vi "Main.vi"() -> ()   [LabVIEW 2015]
doc: "This template is for the Queued Message Handler design pattern.\n\nThe Event Handling Loop generates messages based on user interface actions.\n\nThe Message Handling Loop processes messages generated by the Event Handling Loop, or by other messages. The messages are string values, so new messages can be added easily to the Message Cases case structure in the Message Handling Loop. Each message cluster can also provide an optional value for Message Data, which is a variant that can be converted to whatever message-specific data is required."
uses:
  support/Type Definitions/UI Data.ctl
  support/Status Logger/Status Log.ctl
  <vilib>/Utility/error.llb/DialogType.ctl
  DAQ/TypeDefs/DAQ data.ctl
  support/Message Queue/Enqueue Message (Single).vi
  support/Global names.vi
  <vilib>/Utility/error.llb/Error Cluster From Error Code.vi
  <vilib>/ErrorRing/Error Ring.xnode
  support/Message Queue/Message Queue.lvlib
  Support/User Event - EHL Stop/User Event - EHL Stop.lvlib
  Model/Model.lvlib
  DAQ/DAQ.lvlib
  PLC/PLC.lvlib
panel:
  out "Power status":bool
  in  "Remote":bool
  in  "Abort":bool
  in  "Stop Line":bool
  in  "Start Line":bool
  out "Status":string
  in  "Tab Control":T1(tab)
  in  "Power switch":bool
  in  "Positon":dbl(slide) scale=0.0..20.0
  in  "Dispose":bool
  in  "Pump":bool
  in  "Flow [l/s]":dbl=10.0
  in  "Potentiometer (AI)":tag
  in  "LED (DO)":tag
  in  "Bistable switch (DI)":tag
  in  "Monostable switch (DI)":tag
  in  "Send":bool
  in  "Data to send":string
  out "Data received":string
  in  "Disconnect":bool
  in  "Connect":bool
  out "Connected?":bool
  in  "Type":enum16{"Server", "Client"}(ring)
  in  "Port":u16
  in  "IP":string
  in  "Current printer":u16(ring) items=["PDFCreator", "OKI DATA CORP C5950 kolor (C-2 218)", "Microsoft XPS Document Writer", "Microsoft Print to PDF", "HP LaserJet Professional P1606dn B&W (M3)", "hp LaserJet 1320 PCL 5 B&W (C-2 307)", "Fax", "Canon MP560 KOLOR (DOM)", "Brother PC-FAX v.3.2", "Brother MFC-L8850CDW KOLOR (M6)", "Brother MFC-L2740DW B&W (M6)", "Brother MFC-L2740DW B&W (M3)", "Brother DCP-9020CDW (Dziekan)"]
  in  "Check printers":bool
  in  "Print report":bool
  in  "TDMS View":bool
  in  "Exit":bool
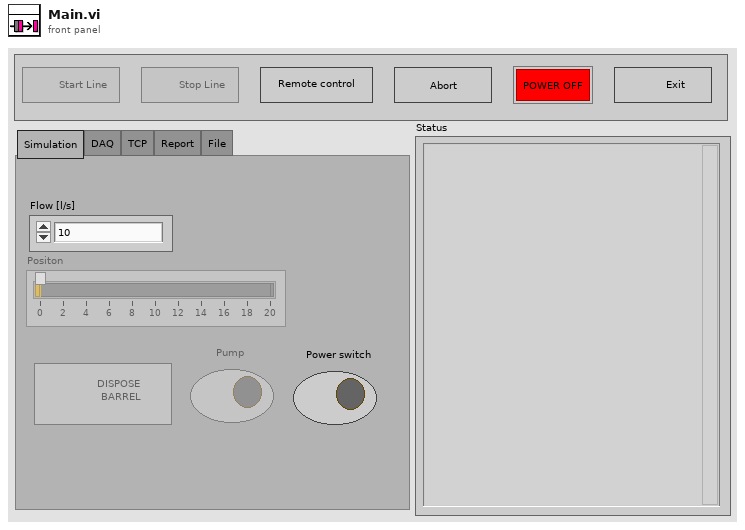
[diagram p1: front panel]
types:
  T1 = enum32{"Simulation", "DAQ", "TCP", "Report", "File"}
  T2 = typedef "Status Log.ctl" = enum16{"Close file", "Open Status file", "Add Status", "Show Status File"}
  T3 = typedef "UI Data.ctl" = cluster{"Start Line Ref":refnum<vi>, "Stop Line Ref":refnum<vi>, "Data Display Ref":refnum<vi>, "Exit Button Ref":refnum<vi>, "Pump Ref":refnum<vi>, "Dispose Ref":refnum<vi>, "Flow Ref":refnum<vi>, "Position Ref":refnum<vi>, "Tab Ref":refnum<vi>, "Print report":refnum<vi>, "Remote":refnum<vi>, "Connection status":refnum<vi>, "Abort":refnum<vi>, "Power status":refnum<vi>, "Power switch":refnum<vi>}
  T4 = typedef "Notifiers.lvlib/Notifiers.ctl" = cluster{"PLC":refnum<notifier>, "Model":refnum<notifier>, "DAQ":refnum<notifier>}
  T5 = typedef "Message Queue.lvlib/All Message Queues.ctl" = cluster{"UI":refnum<queue>, "Model":refnum<queue>, "DAQ":refnum<queue>, "PLC":refnum<queue>}
  T6 = typedef "DialogType.ctl" = u16
  T7 = typedef "DAQ.lvlib/DAQ data.ctl" = cluster{"Power switch (DI)":cluster{"Channel":tag, "Data":bool}, "Dispose barrel (DI)":cluster{"Channel":tag, "Data":bool}, "Pump status (DO)":cluster{"Channel":tag, "Data":bool}, "Barrel position (AI)":cluster{"Channel":tag, "Data":dbl}}
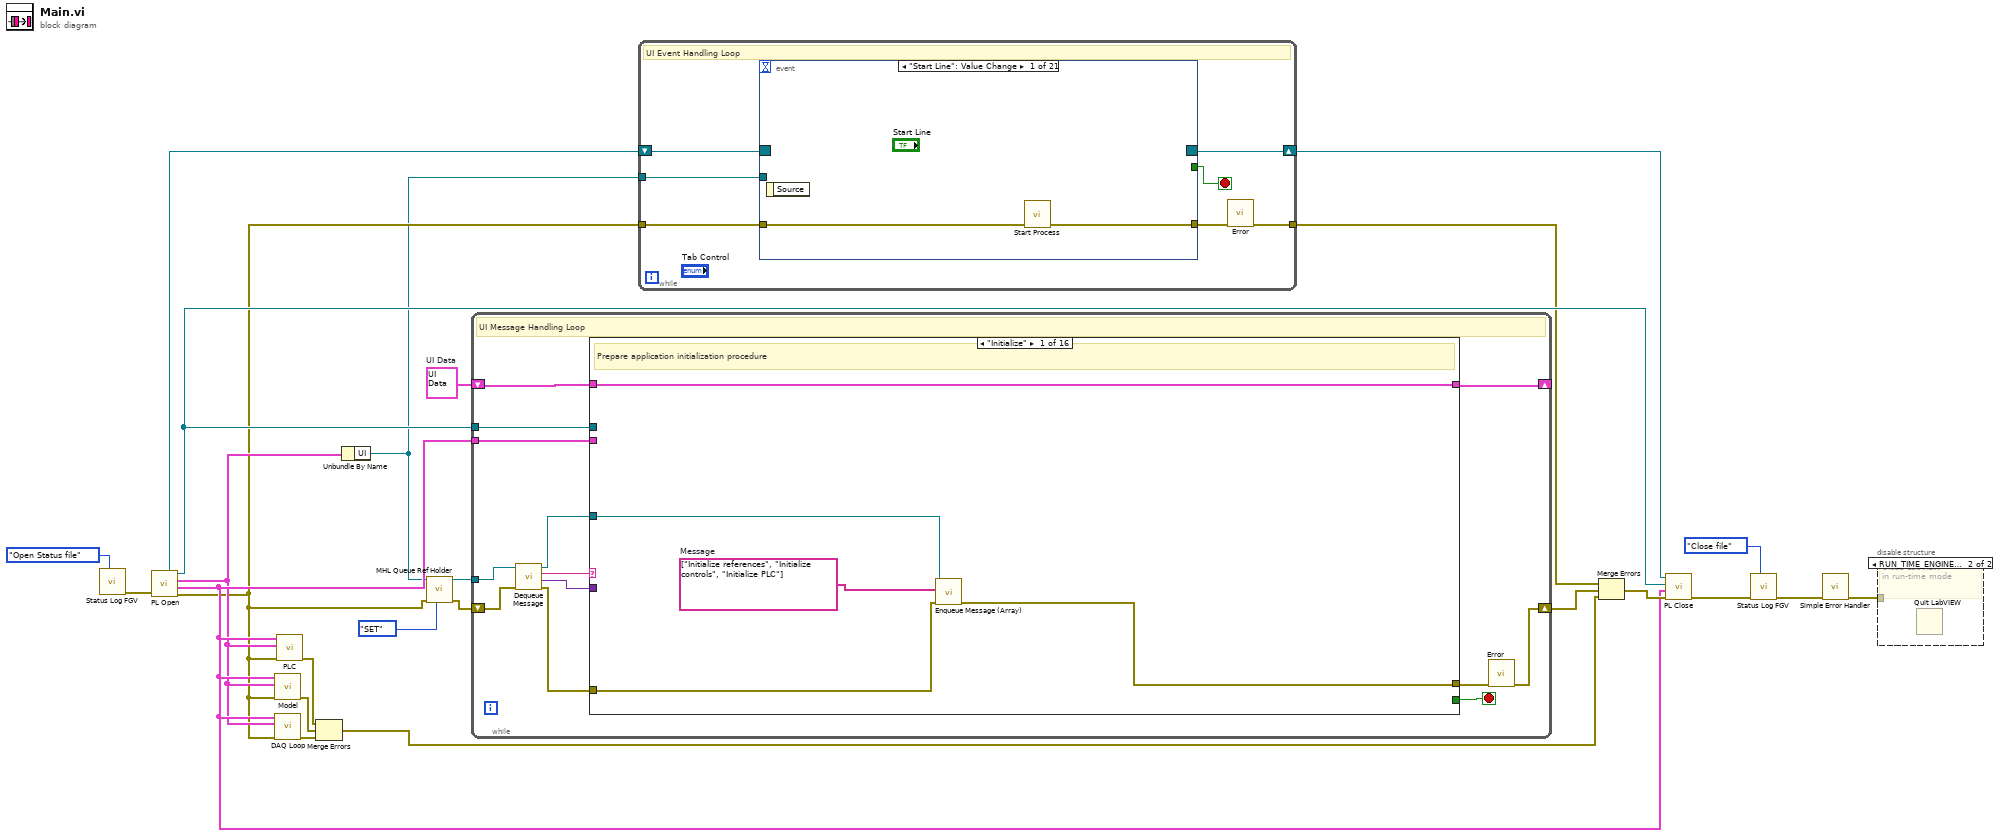
[diagram p0: block diagram]
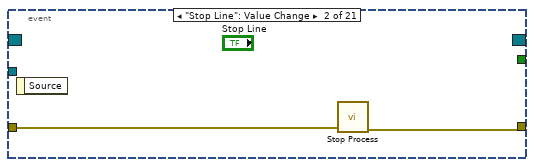
[diagram p2: hidden frame]
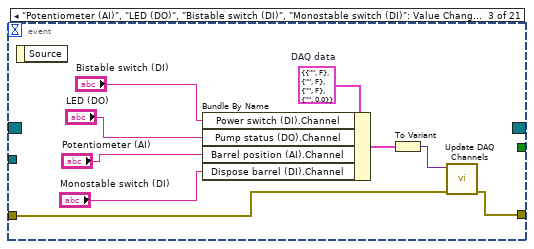
[diagram p3: hidden frame]
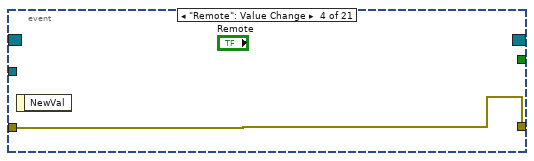
[diagram p4: hidden frame]
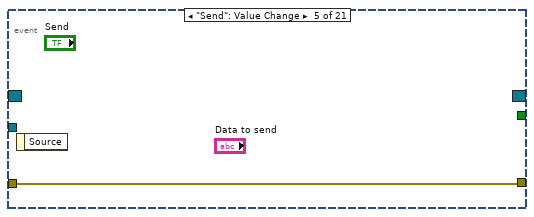
[diagram p5: hidden frame]
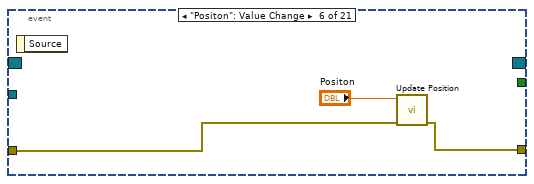
[diagram p6: hidden frame]
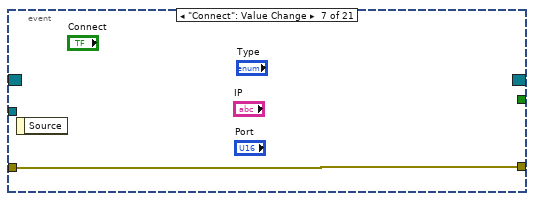
[diagram p7: hidden frame]
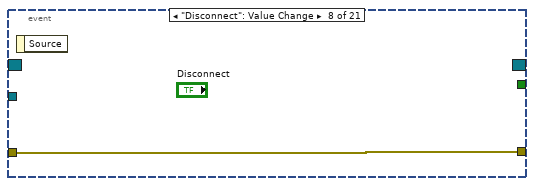
[diagram p8: hidden frame]
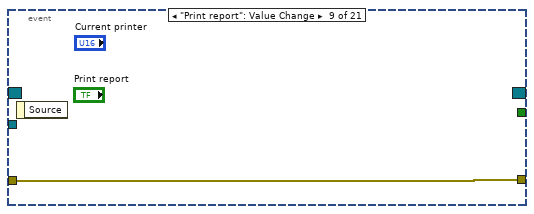
[diagram p9: hidden frame]
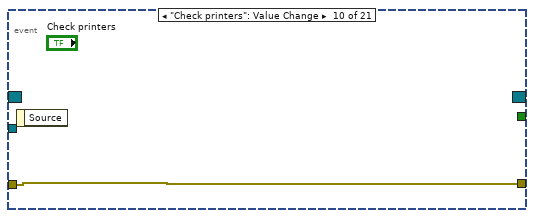
[diagram p10: hidden frame]
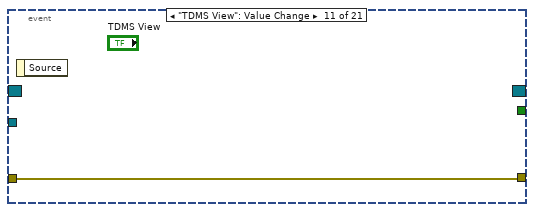
[diagram p11: hidden frame]
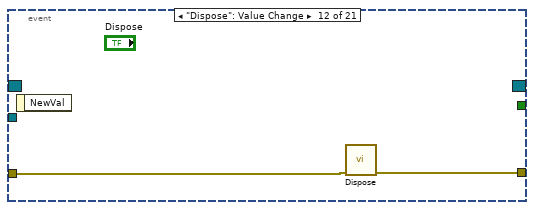
[diagram p12: hidden frame]
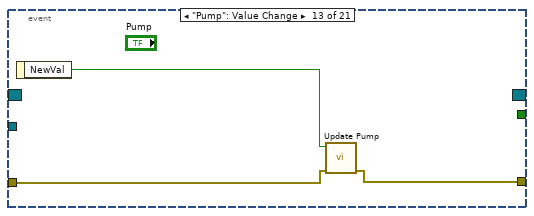
[diagram p13: hidden frame]
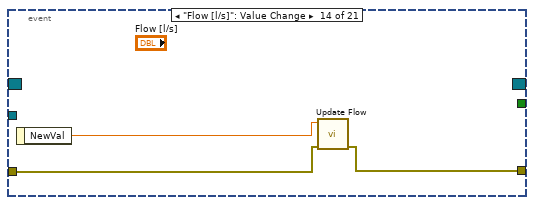
[diagram p14: hidden frame]
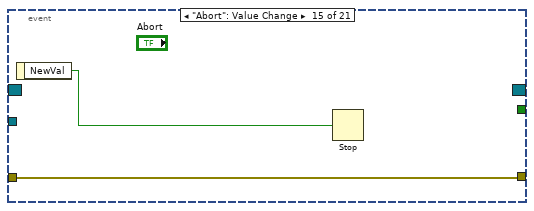
[diagram p15: hidden frame]
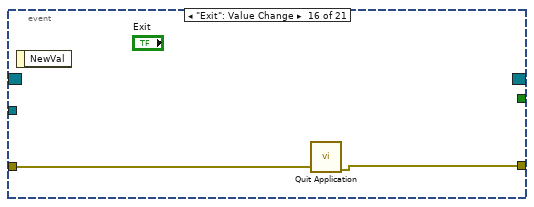
[diagram p16: hidden frame]
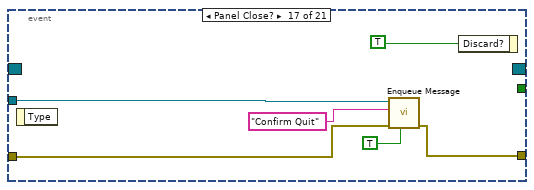
[diagram p17: hidden frame]
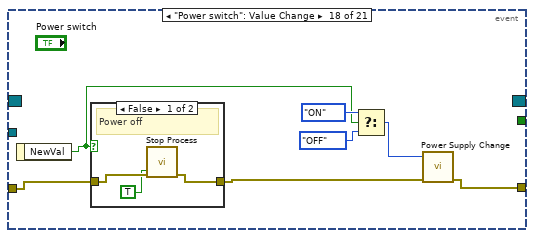
[diagram p18: hidden frame]
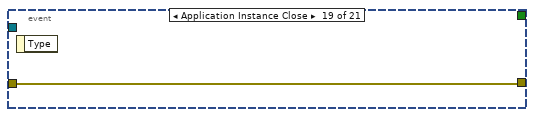
[diagram p20: hidden frame]
diagram:
  w23 = T3 {"Start Line Ref"=refnum, "Stop Line Ref"=refnum, "Data Display Ref"=refnum, "Exit Button Ref"=refnum, "Pump Ref"=refnum, "Dispose Ref"=refnum, "Flow Ref"=refnum, "Position Ref"=refnum, "Tab Ref"=refnum, "Print report"=refnum, "Remote"=refnum, "Connection status"=refnum, "Abort"=refnum, "Power status"=refnum, "Power switch"=refnum}  # UI Data
  n1 = call "Status Log FGV.vi"("Action"=Status_Log."Open Status file") -> ("error out"=w18:errorcluster)  [unwired: 10 in]
  n2 = call "PL Open.vi"("error in"=w18) -> ("error out"=w4:errorcluster, "Notifiers"=w11:T4, "Queues"=w10:T5, "User Event"=w21:refnum<user-event>, "Event Registration Refnum"=w13:refnum<event-registration>)  [unwired: 6 in]
  n3 = call "Model.vi"("error in"=w4, "Queues"=w10, "Notifiers"=w11) -> ("error out"=w8:errorcluster)  [unwired: 8 in]
  n4 = call "DAQ Loop.vi"("error in"=w4, "Queues"=w10, "Notifiers"=w11) -> ("error out"=w7:errorcluster)  [unwired: 8 in]
  n5 = call "PLC.vi"("error in"=w4, "Message Queues"=w10, "Notifiers"=w11) -> ("error out"=w9:errorcluster)  [unwired: 8 in]
  n6 = Merge Errors(w9, w8, w7) -> (w6:errorcluster)
  n7 = Unbundle By Name(w10) -> ("UI"=w1:refnum<queue>)
  n8 = call "MHL Queue Ref Holder.vi"("Action"=enum16{"GET", "SET"}."SET", "error in"=w4, "Message Queue In"=w1) -> ("error out"=w3:errorcluster, "Input Message Queue"=w5:refnum<queue>)  [unwired: 7 in]
  n9 = while {
    shift-right: [w36] -> _
    shift-left: w23 -> [w37]
    tunnel: w21 -> [w34]
    tunnel: w11 -> [w30]
    shift-right: [w26] -> w17
    shift-left: w3 -> [w33]
    tunnel: w5 -> [w28]
    stop <- w35 stop-if-true
    # "UI Message Handling Loop"
    n10 = call "Dequeue Message.vi"("error in (no error)"=w33, "Message Queue"=w28) -> ("error out"=w32:errorcluster, "Message Data"=w29:variant, "Message"=w25:string, "dup Message Queue"=w31:refnum<queue>)  [unwired: 6 in]
    n11 = case "Message Cases" shown="\"Initialize\"" w25 {
      selector: w25 -> [_ _ _ _ _ _ _ _ _ _ _ _ _ _ _ w268]
      tunnel: w31 -> [w39 _ _ _ _ _ _ _ _ _ _ w214 w220 w256 _ _]
      tunnel: w32 -> [w40 w46 w69 w103 w118 w137 w151 w167 w174 w203 w206 w215 w222 w239 w263 _]
      tunnel: [w38 w46 w78 w104 w117 w139 w152 w168 w174 w199 w205 w212 w219 w243 w257 w267] -> w27
      tunnel: w37 -> [w41 w60 w89 w105 w124 w149 w158 w171 w175 w181 w210 w216 w226 w248 w262 w269]
      tunnel: [w41 w47 w89 w105 w124 w149 w158 w171 w175 w181 w210 w216 w226 w248 w262 w269] -> w36
      tunnel: [_ _ _ _ _ _ _ _ _ _ _ _ _ TRUE _ _] -> w35
      tunnel: w29 -> [_ _ _ _ _ _ w162 w165 _ w202 w209 _ _ w250 _ _]
      tunnel: w34 -> [_ _ _ _ _ _ _ _ _ _ _ _ _ w253 _ _]
      tunnel: w30 -> [_ _ _ _ _ _ _ _ _ _ _ _ w225 _ _ _]
      frame "Initialize" {
        w42 = string[] ["Initialize references", "Initialize controls", "Initialize PLC"]  # Message
        # "Prepare application initialization procedure"
        n12 = call "Enqueue Message (Array).vi"("error in (no error)"=w40, "Message Array"=w42, "Message Queue"=w39) -> ("error out"=w38:errorcluster)  [unwired: 7 in, 1 out]
      }
      frame "Initialize references" {
        # "Link references to UI objects"
        n13 = control-ref of="Power switch"() -> (w43:refnum<vi>)
        n14 = control-ref of="Stop Line"() -> (w57:refnum<vi>)
        n15 = control-ref of="Flow [l/s]"() -> (w54:refnum<vi>)
        n16 = control-ref of="Dispose"() -> (w55:refnum<vi>)
        n17 = control-ref of="Exit"() -> (w59:refnum<vi>)
        n18 = control-ref of="Start Line"() -> (w58:refnum<vi>)
        n19 = control-ref of="Pump"() -> (w56:refnum<vi>)
        n20 = Bundle By Name(cluster=w60, "Exit Button Ref"=w59, "Start Line Ref"=w58, "Stop Line Ref"=w57, "Pump Ref"=w56, "Dispose Ref"=w55, "Flow Ref"=w54, "Power switch"=w43) -> (w53:T3)
        n21 = control-ref of="Tab Control"() -> (w51:refnum<vi>)
        n22 = control-ref of="Remote"() -> (w49:refnum<vi>)
        n23 = control-ref of="Connection status"() -> (w48:refnum<vi>)
        n24 = control-ref of="Positon"() -> (w52:refnum<vi>)
        n25 = control-ref of="Print report"() -> (w50:refnum<vi>)
        n26 = control-ref of="Power status"() -> (w44:refnum<vi>)
        n27 = control-ref of="Abort"() -> (w45:refnum<vi>)
        n28 = Bundle By Name(cluster=w53, "Position Ref"=w52, "Tab Ref"=w51, "Print report"=w50, "Remote"=w49, "Connection status"=w48, "Abort"=w45, "Power status"=w44) -> (w47:T3)
      }
      frame "Initialize controls" {
        w61 = TRUE ("Enabled")
        w62 = FALSE ("Enabled")
        # "Initialize activity and values of UI objects"
        n29 = Unbundle By Name(w89) -> ("Stop Line Ref"=w102:refnum<vi>, "Print report"=w84:refnum<vi>)
        n30 = Current VI's Menubar() -> (w64:refnum<k9>)
        n31 = Build Array(w102, w84) -> (w101:refnum<vi>[])
        n32 = call "Enable Multiple Controls.vi"("error in"=w69, "Enabled"=w62, "References"=w101) -> ("error out"=w98:errorcluster)  [unwired: 8 in]
        n33 = Set Menu Item Info(7:"Stop" ("item tag"), 8:w69, 9:w62, 11:w64) -> (0:w67:errorcluster, 3:w63:refnum<k9>)  [unwired: 3 in]
        n34 = Unbundle By Name(w89) -> ("Exit Button Ref"=w100:refnum<vi>, "Start Line Ref"=w99:refnum<vi>)
        n35 = call "Power Supply Change.vi"("error in"=w69, "Power status"=enum16{"OFF", "ON"}."OFF") -> ("error out"=w75:errorcluster)  [unwired: 9 in]
        n36 = Build Array(w100, w99) -> (w97:refnum<vi>[])
        n37 = call "Enable Multiple Controls.vi"("error in"=w98, "Enabled"=w61, "References"=w97) -> ("error out"=w92:errorcluster)  [unwired: 8 in]
        n38 = Set Menu Item Info(7:"Start" ("item tag"), 8:w67, 9:w61, 11:w63) -> (0:w65:errorcluster)  [unwired: 3 in, 1 out]
        n39 = Unbundle By Name(w89) -> ("Exit Button Ref"=w96:refnum<vi>, "Start Line Ref"=w95:refnum<vi>, "Stop Line Ref"=w94:refnum<vi>, "Pump Ref"=w93:refnum<vi>, "Remote"=w83:refnum<vi>, "Connection status"=w82:refnum<vi>, "Abort"=w81:refnum<vi>, "Power status"=w80:refnum<vi>, "Power switch"=w71:refnum<vi>)
        n40 = call "Status Display.vi"("Action"=enum16{"Update", "Clear"}."Clear", "error in"=w75) -> ("error out"=w74:errorcluster, "Status"=w72:string)  [unwired: 8 in]
        n41 = local write "Status"(w72) -> ()
        n42 = Build Array(w96, w95, w94, w93, w83, w82, w81, w80, w71) -> (w90:refnum<vi>[])
        n43 = call "Value Multiple Boolean Controls.vi"("error in"=w92, "Value"=FALSE ("Enabled"), "References"=w90) -> ("error out"=w88:errorcluster)  [unwired: 8 in]
        n44 = Unbundle By Name(w89) -> ("Position Ref"=w87:refnum<vi>)
        n45 = Build Array(w87) -> (w86:refnum<vi>[])
        n46 = call "Value Multiple Numeric Controls.vi"("error in"=w88, "Value"=0.0, "References"=w86) -> ("error out"=w77:errorcluster)  [unwired: 8 in]
        n47 = call "Update Display.vi"("error in"=w77, "Message string"="UI initialized") -> ("error out"=w66:errorcluster)  [unwired: 9 in]
        n48 = Merge Errors(w66, w65, w74) -> (w78:errorcluster)
      }
      frame "Initialize PLC" {
        # "Initialize Production Line Controller"
        n49 = call "Initialize.vi"("error in"=w103) -> ("error out"=w104:errorcluster)  [unwired: 10 in]
      }
      frame "Start process" {
        w109 = TRUE ("Enabled")
        w113 = FALSE ("Enabled")
        # "Starts process: start PLC, open logger file, create reports files, enable/disable UI controls and update status display"
        n50 = Unbundle By Name(w124) -> ("Exit Button Ref"=w106:refnum<vi>, "Start Line Ref"=w119:refnum<vi>, "Stop Line Ref"=w123:refnum<vi>)
        n51 = Build Array(w106, w119) -> (w125:refnum<vi>[])
        n52 = Build Array(w123) -> (w122:refnum<vi>[])
        n53 = call "Start.vi"("error in"=w118) -> ("error out"=w121:errorcluster)  [unwired: 10 in]
        n54 = call "Enable Multiple Controls.vi"("error in"=w118, "Enabled"=w109, "References"=w122) -> ("error out"=w111:errorcluster)  [unwired: 8 in]
        n55 = call "Enable Multiple Controls.vi"("error in"=w118, "Enabled"=w113, "References"=w125) -> ("error out"=w115:errorcluster)  [unwired: 8 in]
        n56 = global read "Global names.vi" "Starting"() -> (w107:string)
        n57 = Current VI's Menubar() -> (w108:refnum<k9>)
        n58 = call "Update Display.vi"("error in"=w121, "Message string"=w107) -> ("error out"=w120:errorcluster)  [unwired: 9 in]
        n59 = Set Menu Item Info(7:"Start" ("item tag"), 8:w115, 9:w113, 11:w108) -> (0:w114:errorcluster)  [unwired: 3 in, 1 out]
        n60 = Set Menu Item Info(7:"Stop" ("item tag"), 8:w111, 9:w109, 11:w108) -> (0:w110:errorcluster)  [unwired: 3 in, 1 out]
        n61 = Merge Errors(w120, w114, w110) -> (w117:errorcluster)
      }
      frame "Stop process" {
        w128 = FALSE ("Enabled")
        w129 = TRUE ("Enabled")
        # "Stops process: stop PLC, close logger file, save and close report files, enable/disable UI controls and update status display"
        n62 = Unbundle By Name(w149) -> ("Exit Button Ref"=w126:refnum<vi>, "Start Line Ref"=w142:refnum<vi>, "Stop Line Ref"=w148:refnum<vi>)
        n63 = call "Stop.vi"("error in"=w137) -> ("error out"=w144:errorcluster)  [unwired: 10 in]
        n64 = Build Array(w148) -> (w138:refnum<vi>[])
        n65 = Build Array(w126, w142) -> (w146:refnum<vi>[])
        n66 = global read "Global names.vi" "Stopping"() -> (w127:string)
        n67 = Build Array (concatenate)(w146, w138) -> (w145:refnum<vi>[])
        n68 = call "Enable Multiple Controls.vi"("error in"=w137, "Enabled"=w129, "References"=w146) -> ("error out"=w134:errorcluster)  [unwired: 8 in]
        n69 = call "Enable Multiple Controls.vi"("error in"=w137, "Enabled"=w128, "References"=w138) -> ("error out"=w141:errorcluster)  [unwired: 8 in]
        n70 = call "Value Multiple Boolean Controls.vi"("error in"=w137, "Value"=FALSE, "References"=w145) -> ("error out"=w140:errorcluster)  [unwired: 8 in]
        n71 = call "Update Display.vi"("error in"=w144, "Message string"=w127) -> ("error out"=w143:errorcluster)  [unwired: 9 in]
        n72 = Current VI's Menubar() -> (w135:refnum<k9>)
        n73 = Set Menu Item Info(7:"Start" ("item tag"), 8:w134, 9:w129, 11:w135) -> (0:w132:errorcluster, 3:w130:refnum<k9>)  [unwired: 3 in]
        n74 = Set Menu Item Info(7:"Stop" ("item tag"), 8:w132, 9:w128, 11:w130) -> (0:w131:errorcluster)  [unwired: 3 in, 1 out]
        n75 = Merge Errors(w143, w131, w141, w140) -> (w139:errorcluster)
      }
      frame "Update display" {
        # "Updates status display, status log file and word report file"
        n76 = Variant To Data(error in=w151, type="", Variant=w162) -> (data=w150:string, error out=w155:errorcluster)
        n77 = call "Status Display.vi"("Action"=enum16{"Update", "Clear"}."Update", "error in"=w155, "Status line"=w150) -> ("error out"=w153:errorcluster, "Status"=→"Status":string)  [unwired: 7 in]
        n78 = call "Status Log FGV.vi"("Action"=Status_Log."Add Status", "error in"=w155, "Status"=w150) -> ("error out"=w154:errorcluster)  [unwired: 8 in]
        n79 = property on="Status" class="Str"("Text.Scroll Position"=-1) -> ()  [unwired: 2 in, 2 out]
        n80 = Merge Errors(w154, w153) -> (w152:errorcluster)
      }
      frame "Update position" {
        # "Programmatically update position of the barrel slider"
        n81 = Variant To Data(error in=w167, type=0.0 ("Value"), Variant=w165) -> (data=w163:dbl, error out=w166:errorcluster)
        n82 = Unbundle By Name(w171) -> ("Position Ref"=w170:refnum<vi>)
        n83 = Build Array(w170) -> (w169:refnum<vi>[])
        n84 = call "Value Multiple Numeric Controls.vi"("error in"=w166, "Value"=w163, "References"=w169) -> ("error out"=w168:errorcluster)  [unwired: 8 in]
      }
      frame "Update Connection UI" {
        # "Updates TCP conection UI indicators"
        "Data received" <- "" ("Data received")
        "Connected?" <- FALSE ("Connected?")
      }
      frame "Power status change" {
        # "Update main switch LED and Start/Stop buttons according to power status change (DAQ DI)"
        n85 = Variant To Data(error in=w203, type=TRUE, Variant=w202) -> (data=w182:bool, error out=w186:errorcluster)
        "Power status" <- w182
        n86 = Unbundle By Name(w181) -> ("Position Ref"=w176:refnum<vi>, "Dispose Ref"=w180:refnum<vi>, "Pump Ref"=w179:refnum<vi>)
        n87 = Unbundle By Name(w181) -> ("Start Line Ref"=w178:refnum<vi>, "Stop Line Ref"=w200:refnum<vi>)
        n88 = Build Array(w176, w180, w179, w178) -> (w177:refnum<vi>[])
        n89 = Build Array(w178) -> (w198:refnum<vi>[])
        n90 = Build Array(w200) -> (w195:refnum<vi>[])
        n91 = Build Array (concatenate)(w198, w195) -> (w197:refnum<vi>[])
        n92 = Current VI's Menubar() -> (w189:refnum<k9>)
        n93 = call "Enable Multiple Controls.vi"("error in"=w186, "Enabled"=w182, "References"=w177) -> ("error out"=w193:errorcluster)  [unwired: 8 in]
        n94 = Set Menu Item Info(7:"Start" ("item tag"), 8:w186, 9:w182, 11:w189) -> (0:w187:errorcluster, 3:w183:refnum<k9>)  [unwired: 3 in]
        n95 = call "Value Multiple Boolean Controls.vi"("error in"=w186, "Value"=FALSE, "References"=w197) -> ("error out"=w192:errorcluster)  [unwired: 8 in]
        n96 = call "Enable Multiple Controls.vi"("error in"=w186, "Enabled"=FALSE, "References"=w195) -> ("error out"=w191:errorcluster)  [unwired: 8 in]
        n97 = Set Menu Item Info(7:"Stop" ("item tag"), 8:w187, 9:FALSE ("enabled"), 11:w183) -> (0:w184:errorcluster)  [unwired: 3 in, 1 out]
        n98 = Merge Errors(w193, w192, w191, w184) -> (w199:errorcluster)
      }
      frame "Error" {
        w204 = T6 2 items=["no dialog", "OK message", "continue or stop message", "OK message + warnings", "continue/stop + warnings"] ("type of dialog (OK msg:1)")
        # "Display error dialog box and quit application"
        n99 = Variant To Data(error in=w206, type=errorcluster {"status"=FALSE, "code"=0, "source"=""} ("error constant"), Variant=w209) -> (data=w207:errorcluster, error out=w205:errorcluster)
        n100 = call <vilib>:"Simple Error Handler.vi"("type of dialog (OK msg:1)"=w204, "error in (no error)"=w207) -> ()  [unwired: 3 in, 5 out]
      }
      frame "Exit" {
        # "Start exit procedure: stop PLC, then send Exit message to PLC and go to PLC confirmation loop"
        n101 = Flush Queue(queue=w214, error in (no error)=w215) -> (error out=w211:errorcluster)  [unwired: 2 out]
        n102 = call "Exit PLC.vi"("error in"=w211) -> ("error out"=w213:errorcluster)  [unwired: 10 in]
        n103 = call "Wait on PLC Exit.vi"("error in"=w213) -> ("error out"=w212:errorcluster)  [unwired: 10 in]
      }
      frame "Wait on PLC exit" {
        # "Wait until PLC shutdown"
        n104 = Unbundle By Name(w225) -> ("PLC"=w224:refnum<notifier>)
        n105 = Wait on Notification(notifier=w224, timeout in ms (-1)=10, error in (no error)=w222) -> (notification=w218:string, timed out?=w221:bool, error out=w217:errorcluster)  [unwired: 1 in, 1 out]
        n106 = case shown="True" w221 {
          tunnel: [w227 w236] -> w219
          tunnel: w217 -> [w228 w233]
          tunnel: w220 -> [_ w234]
          tunnel: w218 -> [_ w229]
          frame True {
            # "Shutdown notification from PLC not received"
            n107 = call "Wait on PLC Exit.vi"("error in"=w228) -> ("error out"=w227:errorcluster)  [unwired: 10 in]
          }
          frame False {
            # "Shutdown notification from PLC received (handshake)"
            n108 = call "Update Display.vi"("error in"=w233, "Message string"=w229) -> ("error out"=w232:errorcluster)  [unwired: 9 in]
            n109 = call "Update Display.vi"("error in"=w232, "Message string"="Application quits" ("Message")) -> ("error out"=w231:errorcluster)  [unwired: 9 in]
            n110 = call-poly "Enqueue Message.vi"("error in (no error)"=w231, "Message"="End program", "Message Queue"=w234) -> ("error out"=w236:errorcluster)  [unwired: 7 in, 1 out]
          }
        }
      }
      frame "End program" {
        # "Shutdown MHL and send exit user event to EHL; reset UI controls"
        n111 = call "Fire User Event - EHL Stop.vi"("error in (no error)"=w239, "User Event - Stop"=w253) -> ("error out"=w238:errorcluster)  [unwired: 9 in]
        n112 = Variant To Data(error in=w239, type=errorcluster {"status"=FALSE, "code"=0, "source"=""} ("error constant"), Variant=w250) -> (data=w251:errorcluster)  [unwired: 1 out]
        n113 = Release Queue(queue=w256, force destroy? (F)=TRUE, error in (no error)=w239) -> (error out=w254:errorcluster)  [unwired: 2 out]
        n114 = call <vilib>:"Simple Error Handler.vi"("error in (no error)"=w251) -> ("error out"=w237:errorcluster)  [unwired: 4 in, 4 out]
        n115 = Merge Errors(w238, w237, w254) -> (w244:errorcluster)
        n116 = Unbundle By Name(w248) -> ("Exit Button Ref"=w247:refnum<vi>, "Abort"=w242:refnum<vi>, "Start Line Ref"=w241:refnum<vi>, "Stop Line Ref"=w240:refnum<vi>)
        n117 = Build Array(w247, w242, w241, w240) -> (w246:refnum<vi>[])
        n118 = call "Value Multiple Boolean Controls.vi"("error in"=w244, "Value"=FALSE, "References"=w246) -> ("error out"=w243:errorcluster)  [unwired: 8 in]
      }
      frame "Confirm Quit" {
        # "Confirm Quit - Message that can confirm whether or not the user wants to exit the application."
        n119 = Two Button Dialog(message="Are you sure?", 1:"Continue" ("F button name (\"Cancel\")"), 2:"Quit" ("T button name (\"OK\")")) -> (T button?=w258:bool)
        n120 = case shown="True" w258 {
          tunnel: w263 -> [w264 w266]
          tunnel: [w264 w265] -> w257
          frame False {
          }
          frame True {
            n121 = call "Quit Application.vi"("error in"=w266) -> ("error out"=w265:errorcluster)  [unwired: 10 in]
          }
        }
      }
      frame Default {
        # "Incorrect message: show error and clear error"
        n122 = xnode "Error Ring"("parameter 0"=w268) -> ("error out"=w267:errorcluster)
      }
    }
    n123 = call "Error.vi"("error in"=w27) -> ("error out"=w26:errorcluster)  [unwired: 10 in]
  }
  n124 = while {
    tunnel: w1 -> [w279]
    shift-right: [w282] -> w24
    shift-left: w13 -> [w283]
    tunnel: [w277] -> w12
    tunnel: w4 -> [w280]
    stop <- w281 stop-if-true
    # "UI Event Handling Loop"
    n125 = event shown="[0] \"Start Line\": Value Change" {
      selector: w283 -> [_ _ _ _ _ _ _ _ _ _ _ _ _ _ _ _ _ _ _ _ _]
      dyn-events: [_ _ _ _ _ _ _ _ _ _ _ _ _ _ _ _ _ _ _ _ _] -> w282
      timeout: _ -> [_ _ _ _ _ _ _ _ _ _ _ _ _ _ _ _ _ _ _ _ _]
      tunnel: [_ _ _ _ _ _ _ _ _ _ _ _ _ _ _ _ _ _ _ TRUE ("Discard?") _] -> w281
      tunnel: w279 -> [_ _ _ _ _ _ _ _ _ _ _ _ _ _ _ _ w324 _ _ _ _]
      tunnel: [w284 w286 w296 w297 w298 w300 w302 w303 w304 w305 w306 w307 w310 w313 w316 w317 w323 w325 w336 w337 w340] -> w278
      tunnel: w280 -> [w285 w287 w295 w297 w298 w299 w302 w303 w304 w305 w306 w308 w311 w314 w316 w318 w319 w327 w336 w337 w339]
      event "Start Line": Value Change {
        n126 = event-data() -> ()  [unwired: 1 in, 1 out]
        n127 = call "Start Process.vi"("error in"=w285) -> ("error out"=w284:errorcluster)  [unwired: 10 in]
      }
      event "Stop Line": Value Change {
        n128 = event-data() -> ()  [unwired: 1 in, 1 out]
        n129 = call "Stop Process.vi"("error in"=w287) -> ("error out"=w286:errorcluster)  [unwired: 10 in]
      }
      event "Potentiometer (AI)", "LED (DO)", "Bistable switch (DI)", "Monostable switch (DI)": Value Change {
        w289 = T7 {"Power switch (DI)"={"Channel"="", "Data"=FALSE}, "Dispose barrel (DI)"={"Channel"="", "Data"=FALSE}, "Pump status (DO)"={"Channel"="", "Data"=FALSE}, "Barrel position (AI)"={"Channel"="", "Data"=0.0}}  # DAQ data
        n130 = event-data() -> ()  [unwired: 1 in, 1 out]
        n131 = Bundle By Name(cluster=w289, "Power switch (DI).Channel"="Bistable switch (DI)", "Pump status (DO).Channel"="LED (DO)", "Barrel position (AI).Channel"="Potentiometer (AI)", "Dispose barrel (DI).Channel"="Monostable switch (DI)") -> (w292:T7)
        n132 = To Variant(anything=w292) -> (Variant=w288:variant)
        n133 = call "Update DAQ Channels.vi"("error in"=w295, "Message Data"=w288) -> ("error out"=w296:errorcluster)  [unwired: 9 in]
      }
      event "Remote": Value Change {
        n134 = event-data() -> ()  [unwired: 1 in, 1 out]
      }
      event "Send": Value Change {
        n135 = event-data() -> ()  [unwired: 1 in, 1 out]
      }
      event "Positon": Value Change {
        n136 = event-data() -> ()  [unwired: 1 in, 1 out]
        n137 = call "Update Position.vi"("error in (no error)"=w299, "Position"="Positon") -> ("error out"=w300:errorcluster)  [unwired: 9 in]
      }
      event "Connect": Value Change {
        n138 = event-data() -> ()  [unwired: 1 in, 1 out]
      }
      event "Disconnect": Value Change {
        n139 = event-data() -> ()  [unwired: 1 in, 1 out]
      }
      event "Print report": Value Change {
        n140 = event-data() -> ()  [unwired: 1 in, 1 out]
      }
      event "Check printers": Value Change {
        n141 = event-data() -> ()  [unwired: 1 in, 1 out]
      }
      event "TDMS View": Value Change {
        n142 = event-data() -> ()  [unwired: 1 in, 1 out]
      }
      event "Dispose": Value Change {
        n143 = event-data() -> ()  [unwired: 1 in, 1 out]
        n144 = call "Dispose.vi"("error in (no error)"=w308) -> ("error out"=w307:errorcluster)  [unwired: 10 in]
      }
      event "Pump": Value Change {
        n145 = event-data() -> ("NewVal"=w309:bool)  [unwired: 1 in]
        n146 = call "Update Pump.vi"("error in (no error)"=w311, "Pump State"=w309) -> ("error out"=w310:errorcluster)  [unwired: 9 in]
      }
      event "Flow [l/s]": Value Change {
        n147 = event-data() -> ("NewVal"=w312:dbl)  [unwired: 1 in]
        n148 = call "Update Flow.vi"("error in (no error)"=w314, "Flow"=w312) -> ("error out"=w313:errorcluster)  [unwired: 9 in]
      }
      event "Abort": Value Change {
        n149 = event-data() -> ("NewVal"=w315:bool)  [unwired: 1 in]
        n150 = Stop(stop? (T)=w315) -> ()
      }
      event "Exit": Value Change {
        n151 = event-data() -> ()  [unwired: 1 in, 1 out]
        n152 = call "Quit Application.vi"("error in"=w318) -> ("error out"=w317:errorcluster)  [unwired: 10 in]
      }
      event Panel Close? {
        n153 = event-data() -> ()  [unwired: 1 in, 1 out]
        n154 = call-poly "Enqueue Message.vi"("Priority Message? (F)"=TRUE, "error in (no error)"=w319, "Message"="Confirm Quit", "Message Queue"=w324) -> ("error out"=w323:errorcluster)  [unwired: 6 in, 1 out]
        n155 = event-data("Discard?"=TRUE) -> ()  [unwired: 1 in, 1 out]
      }
      event "Power switch": Value Change {
        n156 = event-data() -> ("NewVal"=w328:bool)  [unwired: 1 in]
        n157 = case shown="False" w328 {
          tunnel: w327 -> [w334 w335]
          tunnel: [w333 w335] -> w326
          frame False {
            # "Power off"
            n158 = call "Stop Process.vi"("Priority Message? (F)"=TRUE, "error in"=w334) -> ("error out"=w333:errorcluster)  [unwired: 9 in]
          }
          frame True {
            # "Power on"
          }
        }
        n159 = Select(t=enum16{"OFF", "ON"}."ON" ("Power status"), s=w328, f=enum16{"OFF", "ON"}."OFF" ("Power status")) -> (s? t:f=w329:enum16{"OFF", "ON"})
        n160 = call "Power Supply Change.vi"("error in"=w326, "Power status"=w329) -> ("error out"=w325:errorcluster)  [unwired: 9 in]
      }
      event Application Instance Close {
        n161 = event-data() -> ()  [unwired: 1 in, 1 out]
      }
      event User Event {
        n162 = event-data() -> ()  [unwired: 1 in, 1 out]
      }
      event Menu Selection (User) {
        n163 = event-data() -> ("ItemTag"=w341:string)  [unwired: 1 in]
        n164 = case shown="\"Stop\"" w341 {
          tunnel: [w342 w343 w347 w348 w350] -> w340
          tunnel: w339 -> [w342 w344 w346 w349 w351]
          frame Default {
          }
          frame "statuslog" {
            n165 = call "Status Log FGV.vi"("Action"=Status_Log."Show Status File", "error in"=w344) -> ("error out"=w343:errorcluster)  [unwired: 9 in]
          }
          frame "Start" {
            n166 = call "Start Process.vi"("error in"=w346) -> ("error out"=w347:errorcluster)  [unwired: 10 in]
          }
          frame "Stop" {
            n167 = call "Stop Process.vi"("error in"=w349) -> ("error out"=w348:errorcluster)  [unwired: 10 in]
          }
          frame "Exit" {
            n168 = call "Quit Application.vi"("error in"=w351) -> ("error out"=w350:errorcluster)  [unwired: 10 in]
          }
        }
      }
    }
    n169 = call "Error.vi"("error in"=w278) -> ("error out"=w277:errorcluster)  [unwired: 10 in]
  }
  n170 = Merge Errors(w12, w17, w6) -> (w16:errorcluster)
  n171 = call "PL Close.vi"("error in"=w16, "Notifiers"=w11, "User Event"=w21, "Event Registration Refnum in"=w24) -> ("error out"=w22:errorcluster)  [unwired: 7 in]
  n172 = call "Status Log FGV.vi"("Action"=Status_Log."Close file", "error in"=w22) -> ("error out"=w14:errorcluster)  [unwired: 9 in]
  n173 = call <vilib>:"Simple Error Handler.vi"("error in (no error)"=w14) -> ("error out"=w15:errorcluster)  [unwired: 4 in, 4 out]
  n174 = disable-structure shown="RUN_TIME_ENGINE==True" {
    disable-tunnel: w15 -> [_ _]
    frame condition #0 (active) {
    }
    frame condition #1 {
      # "Close LabVIEW\nin run-time mode"
      n175 = Quit LabVIEW() -> ()  [unwired: 1 in]
    }
  }
